vi "SetHold.vi"(8 "error in":errorcluster, 11 "VISA resource name":refnum<visa-resource-name>) -> (0 "error out":errorcluster, 2 "8800 Response":string, 3 "VISA resource name out":refnum<visa-resource-name>)   [LabVIEW 2023, in "Thermotron 8800.lvlib"]
doc: "HOLD\nCommand name: Hold program or manual mode operation\nCommand type: Control\nDescription: Places a running program or test in hold mode.\nSyntax: HOLD\nData type: No data\nQuery example: HOLD\n8800 response: 0 (Places the 8800 in hold mode.)"
uses:
  Thermotron 8800.lvlib
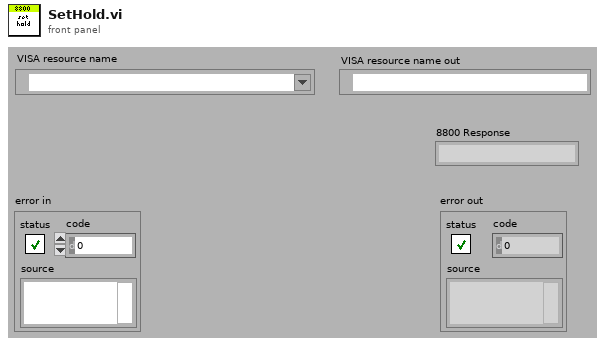
[diagram p1: front panel]
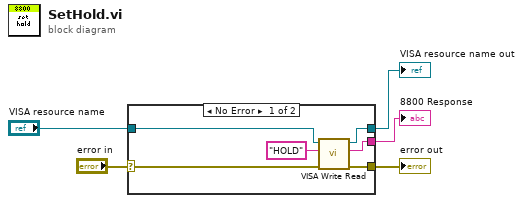
[diagram p0: block diagram]
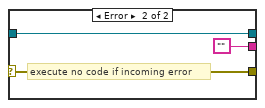
[diagram p2: hidden frame]
diagram:
  n1 = case shown="No Error" "error in" {
    selector: "error in" -> [w10 w14]
    tunnel: [w8 w14] -> w2
    tunnel: [w9 w13] -> w1
    tunnel: "VISA resource name" -> [w11 w13]
    tunnel: [w7 ""] -> w5
    frame No Error {
      n2 = call "VISA Write Read.vi"("error in (no error)"=w10, "8800 Command"="HOLD", "VISA Refnum in"=w11) -> ("error out"=w8:errorcluster, "read buffer"=w7:string, "VISA Refnum out"=w9:refnum<visa-resource-name>)  [unwired: 6 in]
    }
    frame Error {
      # "execute no code if incoming error"
    }
  }
  "VISA resource name out" <- w1
  "error out" <- w2
  "8800 Response" <- w5
